vi "MGCC_Commun_tran_to_global.vi"   [LabVIEW 2016]
uses:
  Model Management/Global_MdlMgmt.vi
  Global communication.vi
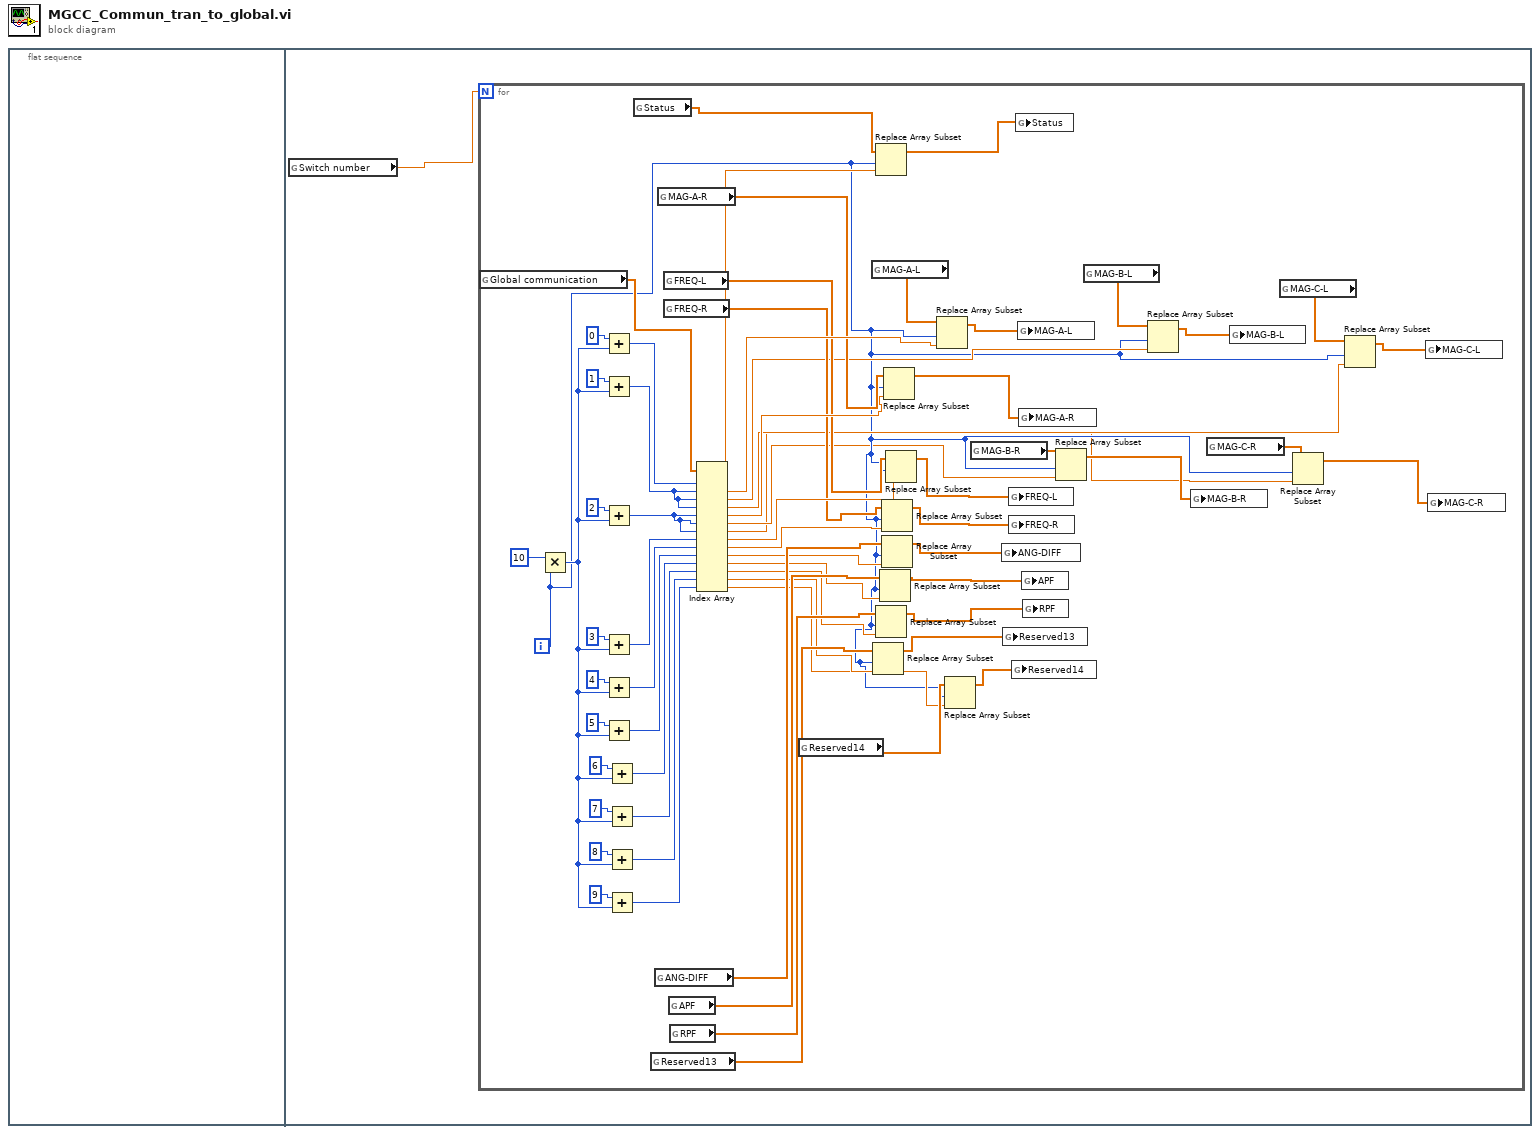
[diagram p0: block diagram]
diagram:
  n1 = flat-sequence {
    frame #0 {
    }
    frame #1 {
      n2 = global read "Global_MdlMgmt.vi" "Switch number"() -> (w1:dbl)
      n3 = for {
        N: w1 -> [_]
        i -> [w4]
        n4 = global read "Global communication.vi" "Global communication"() -> (w48:dbl[])
        n5 = Multiply(x=10, y=w4) -> (x*y=w49:i32)
        n6 = Add(x=0 ("index"), y=w49) -> (x+y=w66:i32)
        n7 = Add(x=1 ("index"), y=w49) -> (x+y=w16:i32)
        n8 = Add(x=2 ("index"), y=w49) -> (x+y=w15:i32)
        n9 = Add(x=3 ("index"), y=w49) -> (x+y=w62:i32)
        n10 = Add(x=4 ("index"), y=w49) -> (x+y=w55:i32)
        n11 = Add(x=5 ("index"), y=w49) -> (x+y=w54:i32)
        n12 = Add(x=6 ("index"), y=w49) -> (x+y=w53:i32)
        n13 = Add(x=7 ("index"), y=w49) -> (x+y=w52:i32)
        n14 = Add(x=8 ("index"), y=w49) -> (x+y=w51:i32)
        n15 = Add(x=9 ("index"), y=w49) -> (x+y=w50:i32)
        n16 = global read "Global communication.vi" "Status"() -> (w46:dbl[])
        n17 = global read "Global communication.vi" "Reserved13"() -> (w21:dbl[])
        n18 = global read "Global communication.vi" "ANG-DIFF"() -> (w30:dbl[])
        n19 = global read "Global communication.vi" "MAG-A-R"() -> (w40:dbl[])
        n20 = global read "Global communication.vi" "FREQ-L"() -> (w37:dbl[])
        n21 = global read "Global communication.vi" "FREQ-R"() -> (w33:dbl[])
        n22 = global read "Global communication.vi" "APF"() -> (w27:dbl[])
        n23 = global read "Global communication.vi" "RPF"() -> (w24:dbl[])
        n24 = Index Array(array=w48, index #1=w66, index #2=w16, index #3=w16, index #4=w16, index #5=w15, index #6=w15, index #7=w15, index #8=w62, index #9=w55, index #10=w54, index #11=w53, index #12=w52, index #13=w51, index #14=w50) -> (element #1=w44:dbl, element #2=w41:dbl, element #3=w10:dbl, element #4=w9:dbl, element #5=w38:dbl, element #6=w3:dbl, element #7=w2:dbl, element #8=w35:dbl, element #9=w32:dbl, element #10=w29:dbl, element #11=w26:dbl, element #12=w23:dbl, element #13=w20:dbl, element #14=w17:dbl)
        n25 = global read "Global communication.vi" "Reserved14"() -> (w18:dbl[])
        n26 = global read "Global communication.vi" "MAG-A-L"() -> (w43:dbl[])
        n27 = Replace Array Subset(array=w21, new element=w20, index=w4) -> (w22:dbl[])
        n28 = Replace Array Subset(array=w46, new element=w44, index=w4) -> (w45:dbl[])
        n29 = Replace Array Subset(array=w24, new element=w23, index=w4) -> (w25:dbl[])
        n30 = Replace Array Subset(array=w27, new element=w26, index=w4) -> (w28:dbl[])
        n31 = Replace Array Subset(array=w33, new element=w32, index=w4) -> (w34:dbl[])
        n32 = Replace Array Subset(array=w30, new element=w29, index=w4) -> (w31:dbl[])
        n33 = Replace Array Subset(array=w40, new element=w38, index=w4) -> (w39:dbl[])
        n34 = Replace Array Subset(array=w37, new element=w35, index=w4) -> (w36:dbl[])
        n35 = Replace Array Subset(array=w43, new element=w41, index=w4) -> (w42:dbl[])
        n36 = Replace Array Subset(array=w18, new element=w17, index=w4) -> (w19:dbl[])
        n37 = global read "Global communication.vi" "MAG-B-R"() -> (w6:dbl[])
        n38 = global write "Global communication.vi" "ANG-DIFF"(w31) -> ()
        n39 = global write "Global communication.vi" "Reserved13"(w22) -> ()
        n40 = global write "Global communication.vi" "FREQ-L"(w36) -> ()
        n41 = global write "Global communication.vi" "FREQ-R"(w34) -> ()
        n42 = global write "Global communication.vi" "Reserved14"(w19) -> ()
        n43 = global write "Global communication.vi" "Status"(w45) -> ()
        n44 = global write "Global communication.vi" "MAG-A-L"(w42) -> ()
        n45 = global write "Global communication.vi" "MAG-A-R"(w39) -> ()
        n46 = global write "Global communication.vi" "APF"(w28) -> ()
        n47 = global write "Global communication.vi" "RPF"(w25) -> ()
        n48 = Replace Array Subset(array=w6, new element=w3, index=w4) -> (w8:dbl[])
        n49 = global read "Global communication.vi" "MAG-B-L"() -> (w14:dbl[])
        n50 = Replace Array Subset(array=w14, new element=w10, index=w4) -> (w13:dbl[])
        n51 = global write "Global communication.vi" "MAG-B-R"(w8) -> ()
        n52 = global read "Global communication.vi" "MAG-C-R"() -> (w5:dbl[])
        n53 = global write "Global communication.vi" "MAG-B-L"(w13) -> ()
        n54 = global read "Global communication.vi" "MAG-C-L"() -> (w12:dbl[])
        n55 = Replace Array Subset(array=w5, new element=w2, index=w4) -> (w7:dbl[])
        n56 = Replace Array Subset(array=w12, new element=w9, index=w4) -> (w11:dbl[])
        n57 = global write "Global communication.vi" "MAG-C-L"(w11) -> ()
        n58 = global write "Global communication.vi" "MAG-C-R"(w7) -> ()
      }
    }
  }
